vi "Get Subscribers.vi"(8 "error in (no error)":errorcluster, 10 "Topic":string, 11 "Broadcaster in":refnum<class "BroadcastBroker.lvclass">) -> (0 "error out":errorcluster, 1 "found":bool, 2 "Subscribers":refnum<class "Message Enqueuer.lvclass">[](array[class]), 3 "Broadcaster out":refnum<class "BroadcastBroker.lvclass">)   [LabVIEW 2019, in "BroadcastBroker.lvclass"]
uses:
  BroadcastBroker.lvclass
  <vilib>/ActorFramework/Message Enqueuer/Message Enqueuer.lvclass
  BroadcastBroker.lvclass/BroadcastBroker.ctl
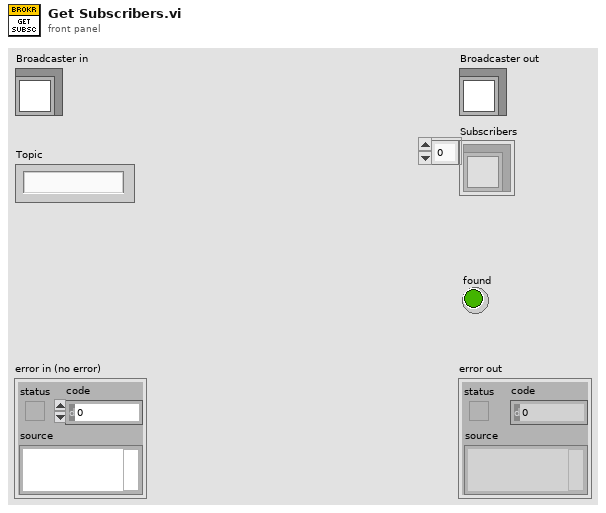
[diagram p1: front panel]
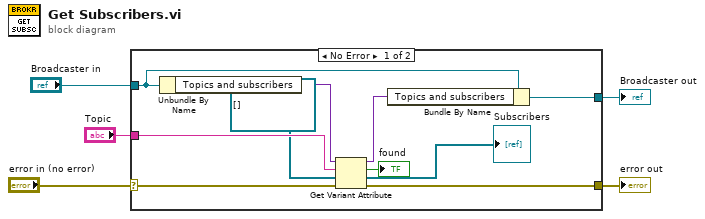
[diagram p0: block diagram]
diagram:
  n1 = case shown="No Error" "error in (no error)" {
    selector: "error in (no error)" -> [w13 w17]
    tunnel: [w11 w17] -> w4
    tunnel: [w9 w16] -> w2
    tunnel: "Broadcaster in" -> [w15 w16]
    tunnel: "Topic" -> [w12 _]
    frame No Error {
      n2 = Unbundle By Name(w15) -> ("Topics and subscribers"=w14:variant)
      n3 = Get Variant Attribute(Variant=w14, name=w12, default value (empty Variant)=refnum<class "Message Enqueuer.lvclass">[] [], error in=w13) -> (duplicate Variant=w10:variant, found=→"found":bool, value=→"Subscribers":refnum<class "Message Enqueuer.lvclass">[], error out=w11:errorcluster)
      n4 = Bundle By Name(cluster=w15, "Topics and subscribers"=w10) -> (w9:refnum<class "BroadcastBroker.lvclass">)
    }
    frame Error {
    }
  }
  "error out" <- w4
  "Broadcaster out" <- w2
